vi "_TangoGroupSize.vi"(2 "error in":errorcluster, 3 "group id":i32) -> (0 "error out":errorcluster, 1 "size":i32)   [LabVIEW 2014, in "tango.lvlib"]
uses:
  tango.lvlib
  tango_binding.so
panel:
  # "Returns the number of devices in the specified group  (i.e. the group size)."
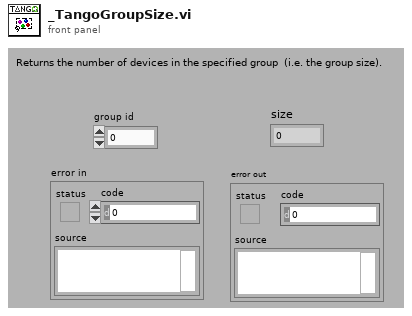
[diagram p1: front panel]
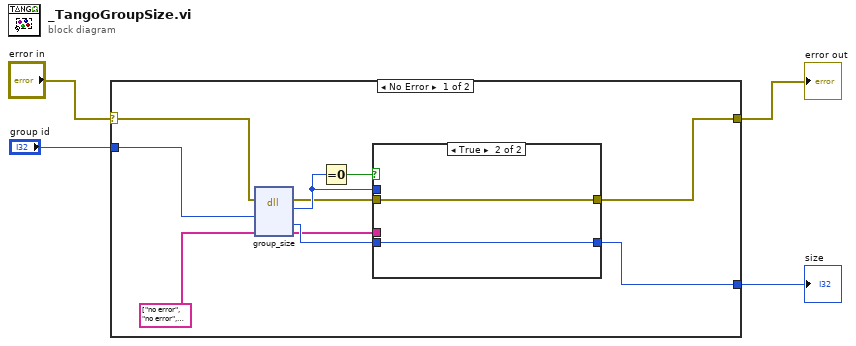
[diagram p0: block diagram]
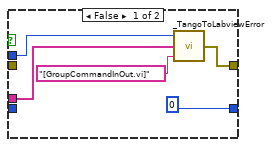
[diagram p2: hidden frame]
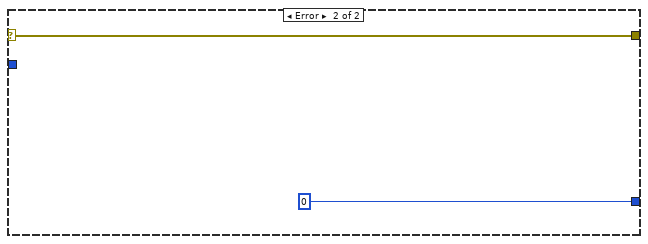
[diagram p3: hidden frame]
diagram:
  n1 = case shown="No Error" "error in" {
    selector: "error in" -> [w12 w23]
    tunnel: "group id" -> [w14 _]
    tunnel: [w5 w23] -> w1
    tunnel: [w9 0 ("size")] -> w2
    frame No Error {
      n2 = dll-call lib="tango_binding.*" fn="group_size"(error in=w12, "group_id"=w14, "error_stack"=string[] ["no error", "no error", "no error", "group_size"] ("error stack")) -> (error out=w6:errorcluster, "type de retour"=w7:i32, "size"=w10:i32, "error_stack"=w8:string[])  [unwired: 4 in, 1 out]
      n3 = Equal To 0?(x=w7) -> (x = 0?=w11:bool)
      n4 = case shown="True" w11 {
        tunnel: w10 -> [_ w21]
        tunnel: [0 ("size") w21] -> w9
        tunnel: w8 -> [w17 _]
        tunnel: w7 -> [w16 _]
        tunnel: w6 -> [_ w20]
        tunnel: [w15 w20] -> w5
        frame False {
          n5 = call "_TangoToLabviewError.vi"("location"="[GroupCommandInOut.vi]", "error stack"=w17, "error code"=w16) -> ("error out"=w15:errorcluster)
        }
        frame True {
        }
      }
    }
    frame Error {
    }
  }
  "error out" <- w1
  "size" <- w2
